vi "Configure Optimum Attenuator for Mixer IMD.vi"(7 "Use Eletronic Attenuator (F)":bool, 8 "error in (no error)":errorcluster, 9 "Frequency offset between F1 and F2":dbl, 10 "Power Level at SA":dbl, 11 "SA-FSW in":refnum<class "SA-FSW.lvclass">) -> (0 "error out":errorcluster, 3 "SA-FSW out":refnum<class "SA-FSW.lvclass">)   [LabVIEW 2020, in "SA-FSW.lvclass"]
uses:
  SA-FSW.lvclass
  C:/Sandbox/Git_Sandbox/WiSpry Test Framework source code (LV20)/WiSpry Test Framework/Instruments/Spectrum Analyzer/Spectrum Analyzer.lvclass
  Spectrum Analyzer.lvclass/Spectrum Analyzer.ctl
  Spectrum Analyzer.lvclass
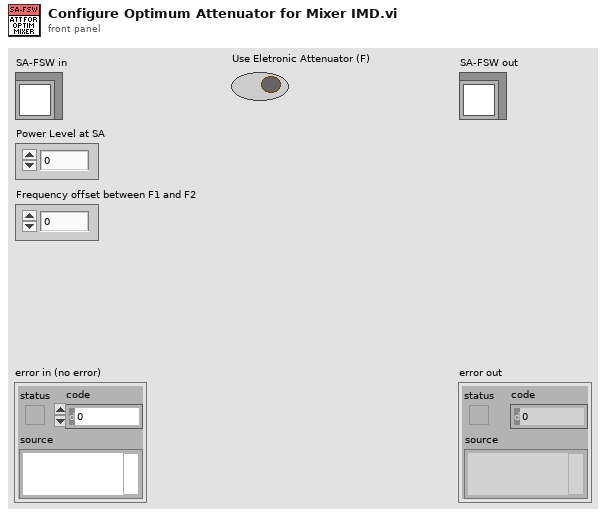
[diagram p1: front panel]
types:
  T1 = cluster{"Offset Frequency":dbl, "Mixer Level":dbl}[]
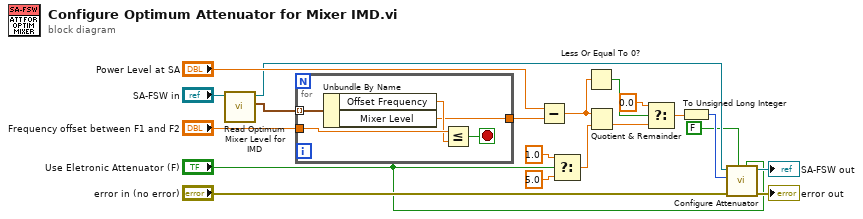
[diagram p0: block diagram]
diagram:
  n1 = call "Read Optimum Mixer Level for IMD.vi"("Spectrum Analyzer in"="SA-FSW in") -> ("Optimum Mixer Level for IMD"=w19:T1, "Spectrum Analyzer out"=w8:refnum<class "SA-FSW.lvclass">)  [unwired: 9 in]
  n2 = for {
    tunnel: w19 -> [w25] mode=indexing
    tunnel: "Frequency offset between F1 and F2" -> [w24]
    tunnel: [w21] -> w16
    stop <- w22 stop-if-true
    n3 = Unbundle By Name(w25) -> ("Offset Frequency"=w23:dbl, "Mixer Level"=w21:dbl)
    n4 = Less Or Equal?(x=w24, y=w23) -> (x <= y?=w22:bool)
  }
  n5 = Subtract(x="Power Level at SA", y=w16) -> (x-y=w10:dbl)
  n6 = Select(t=1.0, s="Use Eletronic Attenuator (F)", f=5.0) -> (s? t:f=w11:dbl)
  n7 = Less Or Equal To 0?(x=w10) -> (x <= 0?=w15:bool)
  n8 = Quotient & Remainder(x=w10, y=w11) -> (floor(x/y)=w9:dbl)  [unwired: 1 out]
  n9 = Select(t=0.0, s=w15, f=w9) -> (s? t:f=w7:dbl)
  n10 = To Unsigned Long Integer(number=w7) -> (unsigned 32bit integer=w6:u32)
  n11 = call-dynamic "Configure Attenuator.vi"("Use Eletronic Attenuator (F)"="Use Eletronic Attenuator (F)", "Auto Attenuator (T)"=FALSE, "error in (no error)"="error in (no error)", "Attenuator (dB)"=w6, "SA-FSW in"=w8) -> ("error out"=→"error out":errorcluster, "SA-FSW out"=→"SA-FSW out":refnum<class "SA-FSW.lvclass">)  [unwired: 5 in]
